vi "Get Device ID.vi"(8 "Error In":errorcluster, 11 "LINX Device Config":T1) -> (0 "Error Out":errorcluster, 1 "Device ID":u8, 2 "Device Family":u8, 3 "LINX Device Config":T1)   [LabVIEW 2011, in "LMH-LINX.lvlib" / "Device.lvlib"]
uses:
  Device.lvlib
  Type Defs/LINX Device Config.ctl
  Type Defs/Interface.ctl
  Type Defs/TCP Config.ctl
  Type Defs/Channels.ctl
  Type Defs/Error Type.ctl
  LMH-LINX.lvlib
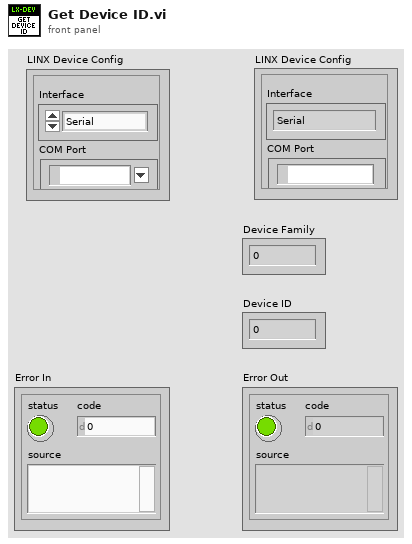
[diagram p1: front panel]
types:
  T1 = typedef "LMH-LINX.lvlib/Device.lvlib/LINX Device Config.ctl" = cluster{"Interface":T2, "COM Port":refnum<visa-resource-name>, "TCP Configuration":T3, "Device Family":u8, "Device ID":u8, "Device Name":string, "TCP Ref":refnum<k5>, "Channels":T4}
  T2 = typedef "LMH-LINX.lvlib/Interface.ctl" = enum16{"Serial", "TCP"}
  T3 = typedef "LMH-LINX.lvlib/Device.lvlib/TCP Config.ctl" = cluster{"IP Address":string, "Port":u16}
  T4 = typedef "LMH-LINX.lvlib/Channels.ctl" = cluster{"DI":u8[], "DO":u8[], "AI":u8[], "AO":u8[], "PWM":u8[], "QE":u8[], "UART":u8[], "I2C 2":u8[], "SPI":u8[], "CAN":u8[], "Servo":u8[], "AI Ref (V)":dbl, "AO Ref (V)":dbl, "AO Resolution (Bits)":u8}
  T5 = typedef "LMH-LINX.lvlib/Error Type.ctl" = enum16{"Unknown", "Timeout", "Corrupt Return Packet", "Unable To Connect", "Command Not Supported", "Channel DNE", "Invalid COM Config", "Firmware Version Mismatch", "myRIO Support", "CMD Specific Error"}
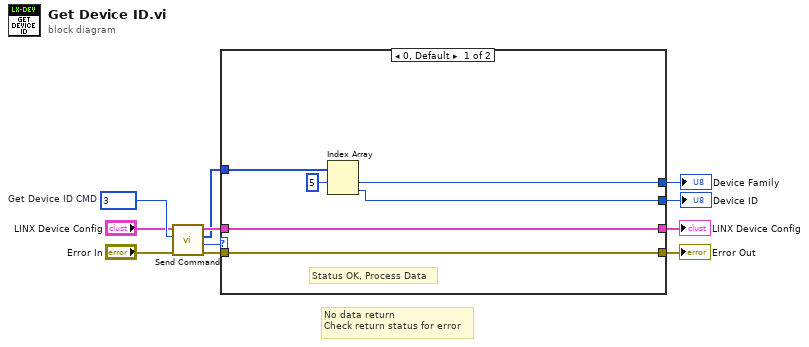
[diagram p0: block diagram]
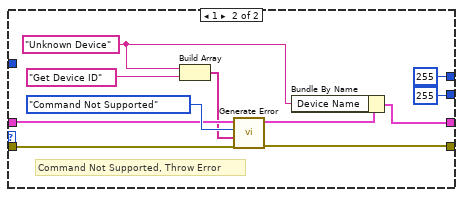
[diagram p2: hidden frame]
diagram:
  w10 = u16 3  # Get Device ID CMD
  # "No data return\nCheck return status for error"
  n1 = call "Send Command.vi"("Error In"="Error In", "CMD"=w10, "LINX Device Config"="LINX Device Config") -> ("Error Out"=w5:errorcluster, "Status"=w3:u8, "Response"=w4:u8[], "LINX Device Config"=w7:T1)  [unwired: 5 in]
  n2 = case shown="0, Default" w3 {
    tunnel: [w15 w21] -> w8
    tunnel: w7 -> [w15 w24]
    tunnel: [w14 w27] -> w6
    tunnel: w5 -> [w14 w28]
    tunnel: w4 -> [w17 _]
    tunnel: [w13 u8 255 ("element")] -> w2
    tunnel: [w12 u8 255 ("element")] -> w1
    frame 0, Default {
      # "Status OK, Process Data"
      n3 = Index Array(array=w17, index #1=5 ("index")) -> (element #1=w13:u8, element #2=w12:u8)  [unwired: 1 in]
    }
    frame 1 {
      w20 = "Unknown Device" ("Device Name")
      # "Command Not Supported, Throw Error"
      n4 = Build Array(w20, "Get Device ID") -> (w23:string[])
      n5 = call "Generate Error.vi"("Error In"=w28, "Arguments"=w23, "Error Type"=Error_Type."Command Not Supported", "LINX Device Config"=w24) -> ("Error Out"=w27:errorcluster, "LINX Device Config"=w22:T1)  [unwired: 6 in]
      n6 = Bundle By Name(cluster=w22, "Device Name"=w20) -> (w21:T1)
    }
  }
  "Error Out" <- w6
  "LINX Device Config" <- w8
  "Device Family" <- w2
  "Device ID" <- w1
